vi "hasPacketIdentifier.vi"(11 "PUBREL in":refnum<class "PUBREL.lvclass">) -> (2 "Has Packet Identifier":bool, 3 "PUBREL out":refnum<class "PUBREL.lvclass">)   [LabVIEW 2013, in "MQTT_Control_Packets.lvlib" / "PUBREL.lvclass"]
uses:
  PUBREL.lvclass
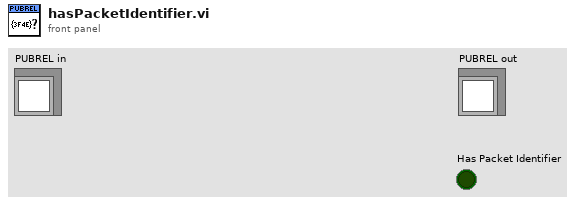
[diagram p1: front panel]
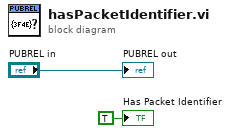
[diagram p0: block diagram]
diagram:
  "PUBREL out" <- "PUBREL in"
  "Has Packet Identifier" <- TRUE ("As Packet Identifier")
